vi "Stop Do.vi"(8 "error in":errorcluster, 11 "Task Actor in":refnum<class "Task Actor.lvclass">) -> (0 "error out":errorcluster, 3 "Task Actor out":refnum<class "Task Actor.lvclass">)   [LabVIEW 2025, in "Task Actor.lvlib" / "Task Actor.lvclass"]
uses:
  Task Actor.lvclass
  <vilib>/ActorFramework/Time-Delayed Send Message/Time-Delay Override Options.ctl
  <vilib>/ActorFramework/Actor/Actor.lvclass/Actor.ctl
  Task Actor.lvclass/Task Actor.ctl
  <vilib>/ActorFramework/Actor/Actor.lvclass
  HAL/MSS/MSS.lvclass
  <vilib>/ActorFramework/Actor Framework.lvlib
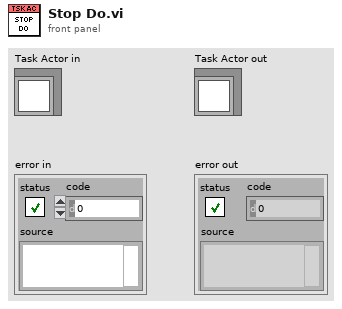
[diagram p1: front panel]
types:
  T1 = typedef "Actor Framework.lvlib/Time-Delay Override Options.ctl" = enum16{"Send next copy now", "Skip next scheduled copy", "Send next copy now and stop all further copies", "Stop all further copies"}
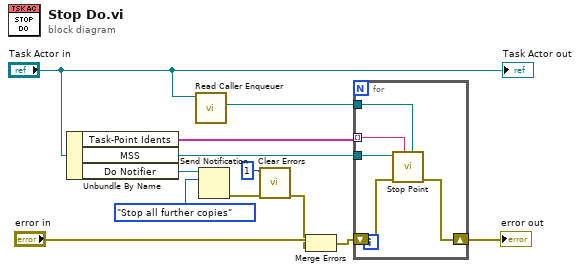
[diagram p0: block diagram]
diagram:
  n1 = Unbundle By Name("Task Actor in") -> ("Task-Point Idents"=w8:string[], "MSS"=w9:refnum<class "MSS.lvclass">, "Do Notifier"=w7:refnum<notifier>)
  n2 = call <vilib>:"Read Caller Enqueuer.vi"("Actor"="Task Actor in") -> ("Caller Enqueuer"=w12:refnum<class "Message Enqueuer.lvclass">)  [unwired: 10 in]
  n3 = Send Notification(notification=Time-Delay_Override_Options."Stop all further copies", notifier=w7) -> (error out=w3:errorcluster)  [unwired: 1 in, 1 out]
  n4 = call <vilib>:"Clear Errors.vi"("error in (no error)"=w3, "specific error code to clear (0: all)"=1) -> ("error out"=w2:errorcluster)  [unwired: 4 in, 1 out]
  n5 = Merge Errors("error in", w2) -> (w4:errorcluster)
  n6 = for {
    tunnel: w9 -> [w17]
    shift-right: [w15] -> w10
    shift-left: w4 -> [w16]
    tunnel: w8 -> [w14] mode=indexing
    tunnel: w12 -> [w13]
    n7 = call "Stop Point.vi"("Series Enqueuer"=w13, "Task-Point Ident"=w14, "error in"=w16, "MSS in"=w17) -> ("error out"=w15:errorcluster)  [unwired: 6 in, 1 out]
  }
  "error out" <- w10
  "Task Actor out" <- "Task Actor in"
